vi "onCreate.vi"(8 "error in (no error)":errorcluster, 11 "Pump":refnum<class "Pump.lvclass">) -> (0 "error out":errorcluster, 3 "Pump out":refnum<class "Pump.lvclass">)   [LabVIEW 2014, in "Pump.lvclass"]
doc: "JKI State Machine Objects (SMO) 1.4.0.57\nJKI - JKI\nCopyright (c) 2018, JKI"
uses:
  Pump.lvclass
  Query Payload -- cluster.ctl
  Pump State - cluster.ctl
  Parameters Payload -- cluster.ctl
  Parameters - cluster.ctl
  Pump.lvclass/Pump.ctl
  <vilib>/JKI/JKI SMO/SMO/SMO.lvclass
panel:
  # "For instructions on how to use the JKI State Machine Objects, examples and video tutorials, visit:\nhttp://jki.net/state-machine-objects/\n\nJKI State Machine Objects™\nhttp://jki.net/state-machine-objects/\nCopyright (C) 2005-2015, JKI <info@jki.net>\nALL RIGHTS RESERVED"
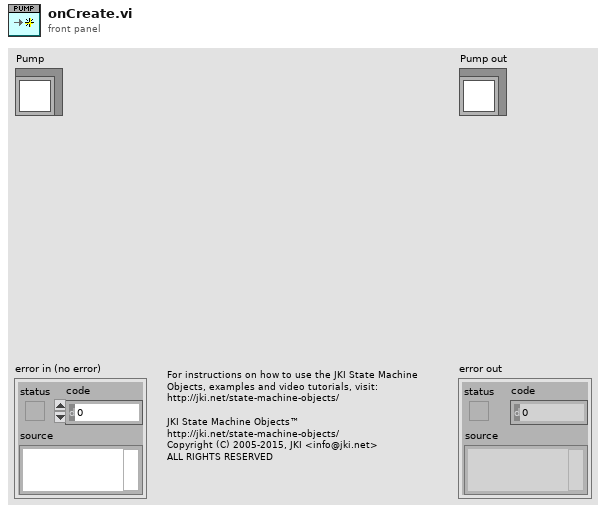
[diagram p1: front panel]
types:
  T1 = typedef "Pump.lvclass/Parameters Payload -- cluster.ctl" = cluster{"Parameters":T2, "notifier":refnum<notifier>}
  T2 = typedef "Pump.lvclass/Parameters - cluster.ctl" = cluster{"Kc":dbl, "Ti":dbl, "Td":dbl, "Min Speed":dbl, "Max Speed":dbl}
  T3 = typedef "Pump.lvclass/Pump State - cluster.ctl" = cluster{"Pump Setpoint":dbl, "Pump Speed":dbl, "Output %":dbl}
  T4 = typedef "Pump.lvclass/Query Payload -- cluster.ctl" = cluster{"value":dbl, "notifier":refnum<notifier>}
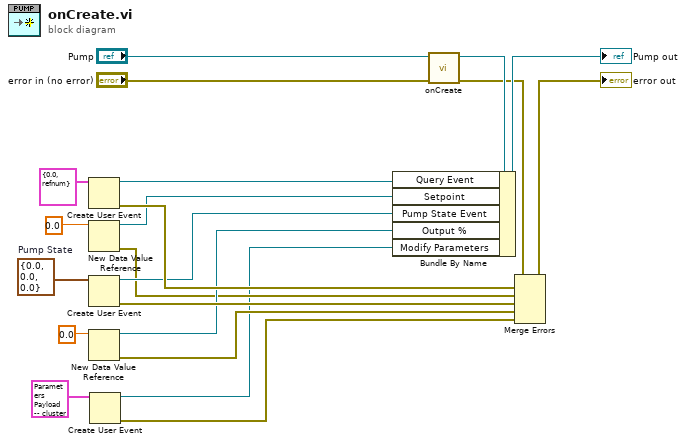
[diagram p0: block diagram]
diagram:
  w10 = T3 {"Pump Setpoint"=0.0, "Pump Speed"=0.0, "Output %"=0.0}  # Pump State
  n1 = Create User Event(user event datatype=T4 {"value"=0.0, "notifier"=refnum} ("Query Payload")) -> (user event=w14:refnum<user-event>, error out=w13:errorcluster)  [unwired: 1 in]
  n2 = New Data Value Reference(data value=0.0 ("Output %")) -> (data value reference=w11:refnum<data-value>, error out=w4:errorcluster)  [unwired: 1 in]
  n3 = Create User Event(user event datatype=w10) -> (user event=w9:refnum<user-event>, error out=w8:errorcluster)  [unwired: 1 in]
  n4 = New Data Value Reference(data value=0.0 ("Output %")) -> (data value reference=w6:refnum<data-value>, error out=w5:errorcluster)  [unwired: 1 in]
  n5 = Create User Event(user event datatype=T1 {"Parameters"={"Kc"=1.0, "Ti"=0.1, "Td"=0.0, "Min Speed"=0.0, "Max Speed"=100.0}, "notifier"=refnum} ("Parameters Payload")) -> (user event=w2:refnum<user-event>, error out=w1:errorcluster)  [unwired: 1 in]
  n6 = call-parent "onCreate.vi"("error in (no error)"="error in (no error)", "SMO"="Pump") -> ("error out"=w17:errorcluster, "SMO out"=w21:refnum<class "Pump.lvclass">)  [unwired: 8 in]
  n7 = Bundle By Name(cluster=w21, "Query Event"=w14, "Setpoint"=w11, "Pump State Event"=w9, "Output %"=w6, "Modify Parameters"=w2) -> (→"Pump out":refnum<class "Pump.lvclass">)
  n8 = Merge Errors(w17, w13, w4, w8, w5, w1) -> (→"error out":errorcluster)
